vi "Build Auth String.vi"(9 "Challenge":string="+IxH4CnCiqpX1rM9scsNynZzbOe4KhDeYcTNS3PDaeY=", 10 "Salt":string="lM1GncleQOaCu9lT1yeUZhFYnqhsLLP1G5lAGo3ixaI=", 11 "Password":string="supersecretpassword") -> (3 "Auth String":string)   [LabVIEW 2020, in "obs-websocket.lvlib" / "OBS.lvclass"]
uses:
  OBS.lvclass
  OBS.lvclass/OBS.ctl
  lv-web-crypto/lv-crypto/Crypto/Hashes/SHA-256/SHA-256.lvclass
  lv-web-crypto/lv-base64/Base64.lvlib
panel:
  out "Challenge Hash":string
  out "Base64 Secret":string
  out "Password + Salt Hash":string
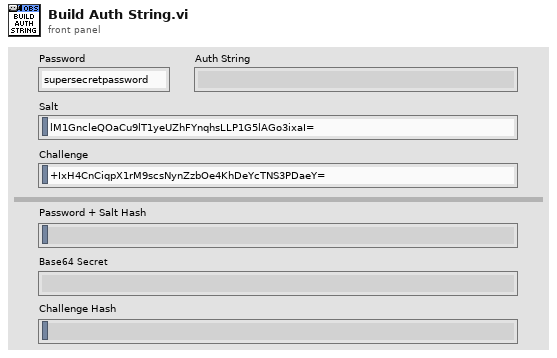
[diagram p1: front panel]
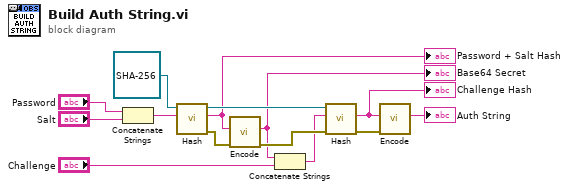
[diagram p0: block diagram]
diagram:
  n1 = Concatenate Strings("Password", "Salt") -> (w1:string)
  n2 = call-dynamic "Hash.vi"("Message"=w1, "SHA-256 in"=refnum<class "SHA-256.lvclass"> refnum ("Crypto.lvlib:SHA-256.lvclass")) -> ("error out"=w8:errorcluster, "Hash"=w3:string, "SHA-256 out"=w5:refnum<class "SHA-256.lvclass">)  [unwired: 7 in]
  "Password + Salt Hash" <- w3
  n3 = call "Encode.vi"("error in (no error)"=w8, "string in (not encoded)"=w3) -> ("error out"=w14:errorcluster, "string out (base64-encoded)"=w4:string)  [unwired: 8 in]
  "Base64 Secret" <- w4
  n4 = Concatenate Strings(w4, "Challenge") -> (w6:string)
  n5 = call-dynamic "Hash.vi"("error in (no error)"=w14, "Message"=w6, "SHA-256 in"=w5) -> ("error out"=w9:errorcluster, "Hash"=w7:string)  [unwired: 6 in, 1 out]
  "Challenge Hash" <- w7
  n6 = call "Encode.vi"("error in (no error)"=w9, "string in (not encoded)"=w7) -> ("string out (base64-encoded)"=→"Auth String":string)  [unwired: 8 in, 1 out]
